vi "Main Loop.vi"(8 "error in (no error)":errorcluster, 10 "Chart Notifier":refnum<notifier>, 11 "Message Queues":T1) -> (0 "error out":errorcluster)   [LabVIEW 2018, in "TCU Module.lvlib" / "TCU Module Engine.lvlib"]
uses:
  TCU Module Engine.lvlib
  All Message Queues.ctl
  support/Message Queue/Message Cluster.ctl
  TCU State Cluster.ctl
  State Enum.ctl
  TCU Module Settings Cluster.ctl
  Output Devices.ctl
  Huber TCU/Huber Settings.ctl
  Lauda Integral XT-150 TCU/Lauda Settings.ctl
  Julabo Type 1 TCU/Julabo Type 1 TCU Folder/Julabo FP-50 Settings.ctl
  Huber Unistat 410 TCU/Huber Unistat 410 Settings.ctl
  TCU Module Display.ctl
  <vilib>/Platform/TimedLoop/XDataNode/timing_clust.ctl
  <vilib>/Platform/TimedLoop/XDataNode/nitl_modes.ctl
  <vilib>/Platform/TimedLoop/XDataNode/wakeup.ctl
  Tag VIs/Tag FGV Operation Enum.ctl
  TCU Module Config Cluster.ctl
  <vilib>/Utility/miscctls.llb/LVPoint32TypeDef.ctl
  support/Message Queue/Enqueue Message (Single).vi
  <vilib>/Platform/TimedLoop/XDataNode/XDataNode.xnode
  support/Message Queue/Message Queue.lvlib
  <vilib>/Platform/TimedLoop/XDataNode/XDNodeRunTimeDep.lvlib
  TCU Module.lvlib
  Shared Variables/Dynamic Shared Variables.lvlib
  Huber TCU/Huber Ministat 230 TCU.lvlib
  Lauda Integral XT-150 TCU/Lauda TCU.lvlib
  Julabo Type 1 TCU/Julabo Type 1 TCU Folder/Julabo Type FP-50 TCU.lvlib
  Huber Unistat 410 TCU/Huber Unistat 410 TCU.lvlib
  support/Support Library.lvlib
panel:
  out "Period (s)":dbl format="%_4g"
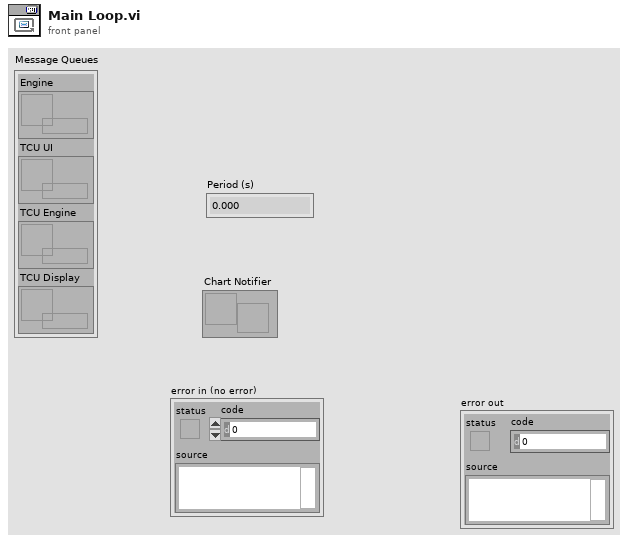
[diagram p1: front panel]
types:
  T1 = typedef "TCU Module.lvlib/All Message Queues.ctl" = cluster{"Engine":refnum<queue>, "TCU UI":refnum<queue>, "TCU Engine":refnum<queue>, "TCU Display":refnum<queue>}
  T2 = typedef "XDNodeRunTimeDep.lvlib/timing_clust.ctl" = cluster{"Expected End [f-1]":u64, "Actual End [f-1]":u64, "Finished Late? [f-1]":bool, "Expected End [i-1]":u64, "Actual End [i-1]":u64, "Finished Late? [i-1]":bool, "Expected Start [i]":u64, "Actual Start [i]":u64, "Expected Start [f]":u64, "Actual Start [f]":u64, "Source Name":string, "Structure Name":string, "Period":i64, "Deadline":i64, "Offset":i64, "Start":i64, "Priority":i32, "Timeout":i32, "Mode":T3, "Wakeup Reason":T4, "Error":errorcluster, "Source Type":string, "Secondary Source Type":string, "Global End Time":u64, "Global Start Time":u64, "Frame Duration":u64, "Iteration Duration":u64, "Assigned CPU":i32, "I/O Scan Engine Mode":u32}
  T3 = typedef "XDNodeRunTimeDep.lvlib/nitl_modes.ctl" = enum32{"No Change", "Process missed periods, maintain original phase", "Discard missed periods, maintain original phase", "Process missed periods, ignore original phase", "Discard missed periods, ignore original phase"}
  T4 = typedef "XDNodeRunTimeDep.lvlib/wakeup.ctl" = enum32{"Normal", "Aborted", "Asynchronous wakeup", "Timing source error", "Timed loop error", "Timeout"}
  T5 = cluster{"enable? (F)":bool, "name":string, "alarm on":bool, "priority":u32, "ack type":enum16{"Auto", "User", "None", "Each Occurrence"}, "area":string, "description":string, "log? (T)":bool}
  T6 = typedef "Tag FGV Operation Enum.ctl" = enum16{"Init", "Set Notification Queue", "Create Tag", "Commit", "Write Tag (Numeric)", "Write Tag (Boolean)", "Read All Tags", "Read One Tag", "Delete Tag Category", "Set Alarm Parameters (Numeric)", "Set Alarm Parameters (Boolean)", "Enable All Alarms", "Disable All Alarms", "Delete All Tags", "Read Alarms", "Ack Alarm", "Read Alarm Parameters (Numeric)", "Read Alarm Parameters (Boolean)"}
  T7 = enum32{"u32BitField", "bool", "double", "string", "int8", "uint8", "int16", "uint16", "int32", "uint32", "int64", "uint64", "single", "double waveform", "int16 waveform", "array of boolean", "array of int8", "array of uint8", "array of int16", "array of uint16", "array of int32", "array of uint32", "array of int64", "array of uint64", "array of single", "array of double", "array of double waveform", "array of int16 waveform", "array of string", "variant", "timestamp", "fixed point", "custom"}
  T8 = typedef "TCU Module.lvlib/TCU Module Engine.lvlib/State Enum.ctl" = enum16{"Measuring", "Idle", "Paused"}
  T9 = typedef "TCU Module.lvlib/TCU Module Config Cluster.ctl" = cluster{"GUID":string, "Drop Coords":T10, "Process Name":string, "Queue Name":string, "Settings":T11, "Load Count":i32, "Power Level Changed":bool}
  T10 = typedef "LVPoint32TypeDef.ctl" = cluster{"Horizontal":i32, "Vertical":i32}
  T11 = typedef "TCU Module.lvlib/TCU Module Settings Cluster.ctl" = cluster{"Cycle Period":dbl, "Setpoint Entry":dbl, "Output Device":T12, "Huber Ministat 230 Settings":T13, "Lauda Settings":T14, "Julabo FP-50 Settings":T15, "Internal Control?":bool, "Huber Unistat 410 Settings":T16}
  T12 = typedef "Output Devices.ctl" = enum16{"Default", "Huber Ministat 230", "Huber Unistat 410", "Lauda XT-150", "Julabo FP-50"}
  T13 = typedef "Huber Ministat 230 TCU.lvlib/Huber Settings.ctl" = cluster{"VISA resource name":refnum<visa-resource-name>, "Simulated?":bool}
  T14 = typedef "Lauda TCU.lvlib/Lauda Settings.ctl" = cluster{"VISA resource name":refnum<visa-resource-name>, "Simulated?":bool, "Pump Power":i32}
  T15 = typedef "Julabo Type FP-50 TCU.lvlib/Julabo FP-50 Settings.ctl" = cluster{"VISA resource name":refnum<visa-resource-name>, "Simulated?":bool, "Pump Power":i32}
  T16 = typedef "Huber Unistat 410 TCU.lvlib/Huber Unistat 410 Settings.ctl" = cluster{"VISA resource name":refnum<visa-resource-name>, "Simulated?":bool}
  T17 = typedef "TCU Module.lvlib/TCU Module Display.ctl" = cluster{"TCU On?":bool, "Cycle Period":dbl, "Current TCU Temp":dbl}
  T18 = typedef "TCU Module.lvlib/TCU Module Engine.lvlib/TCU State Cluster.ctl" = cluster{"State":T8, "Start Time":timestamp, "Configuration":T11, "Current Time":timestamp, "First Iteration":bool, "Data":cluster{"TCU Speed":dbl, "Temperature":dbl}, "Process Name":string, "TCU On?":bool, "Output Error":bool, "Start Log":bool, "Power Level Changed":bool}
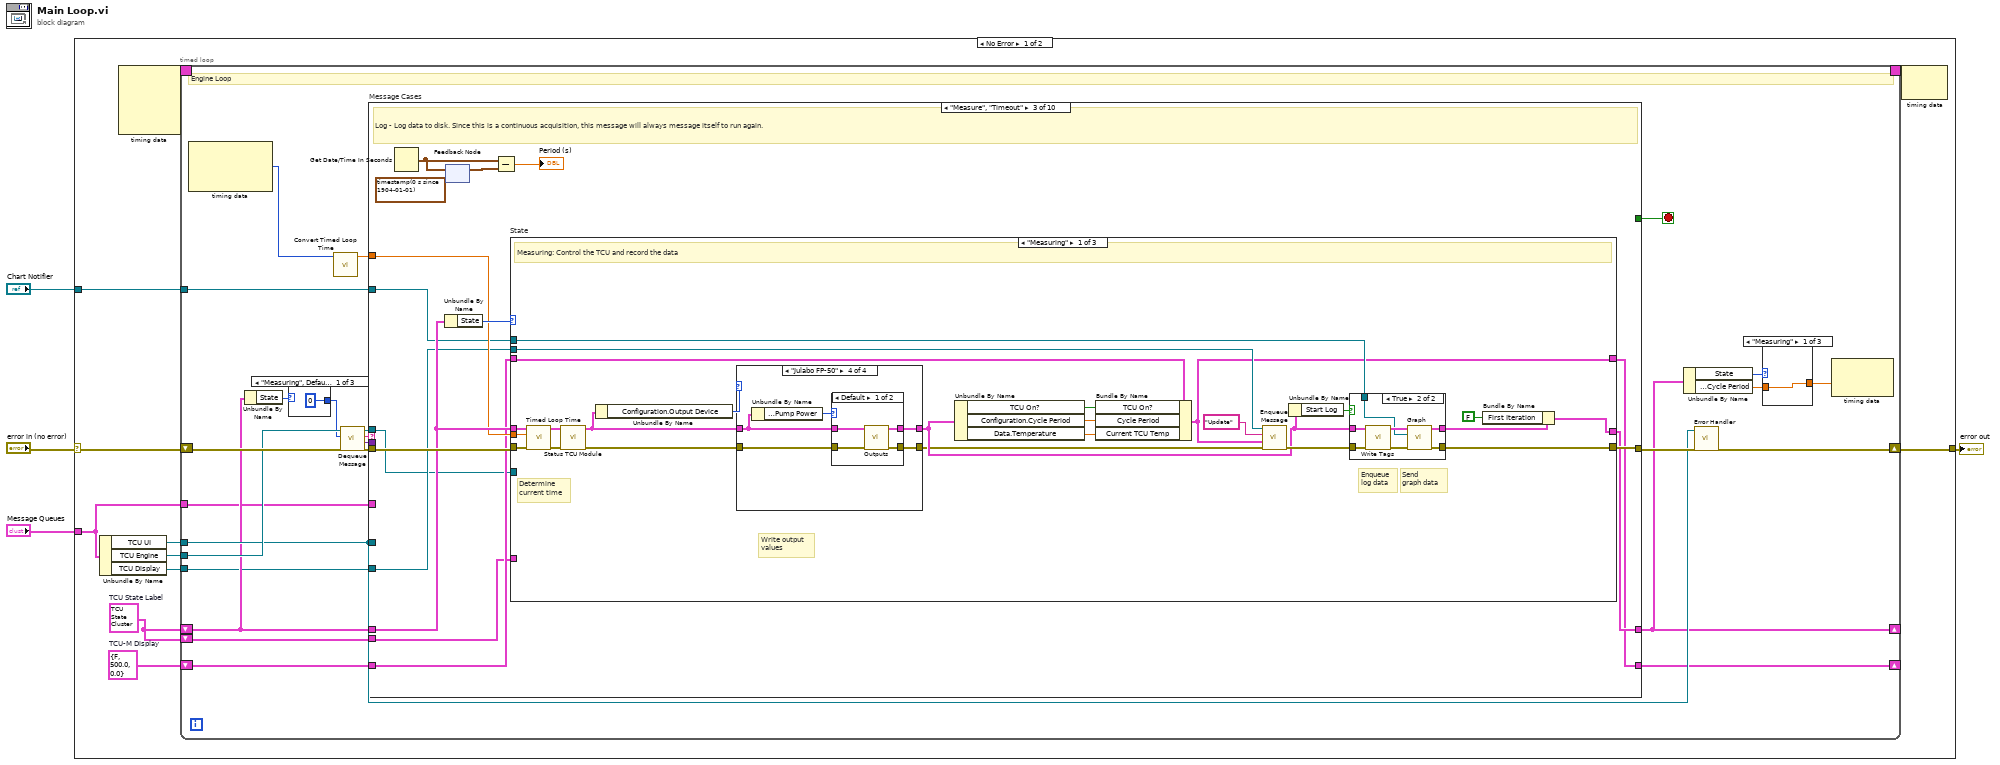
[diagram p0: block diagram]
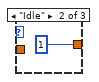
[diagram p2: hidden frame]
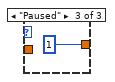
[diagram p3: hidden frame]
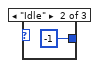
[diagram p4: hidden frame]
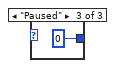
[diagram p5: hidden frame]
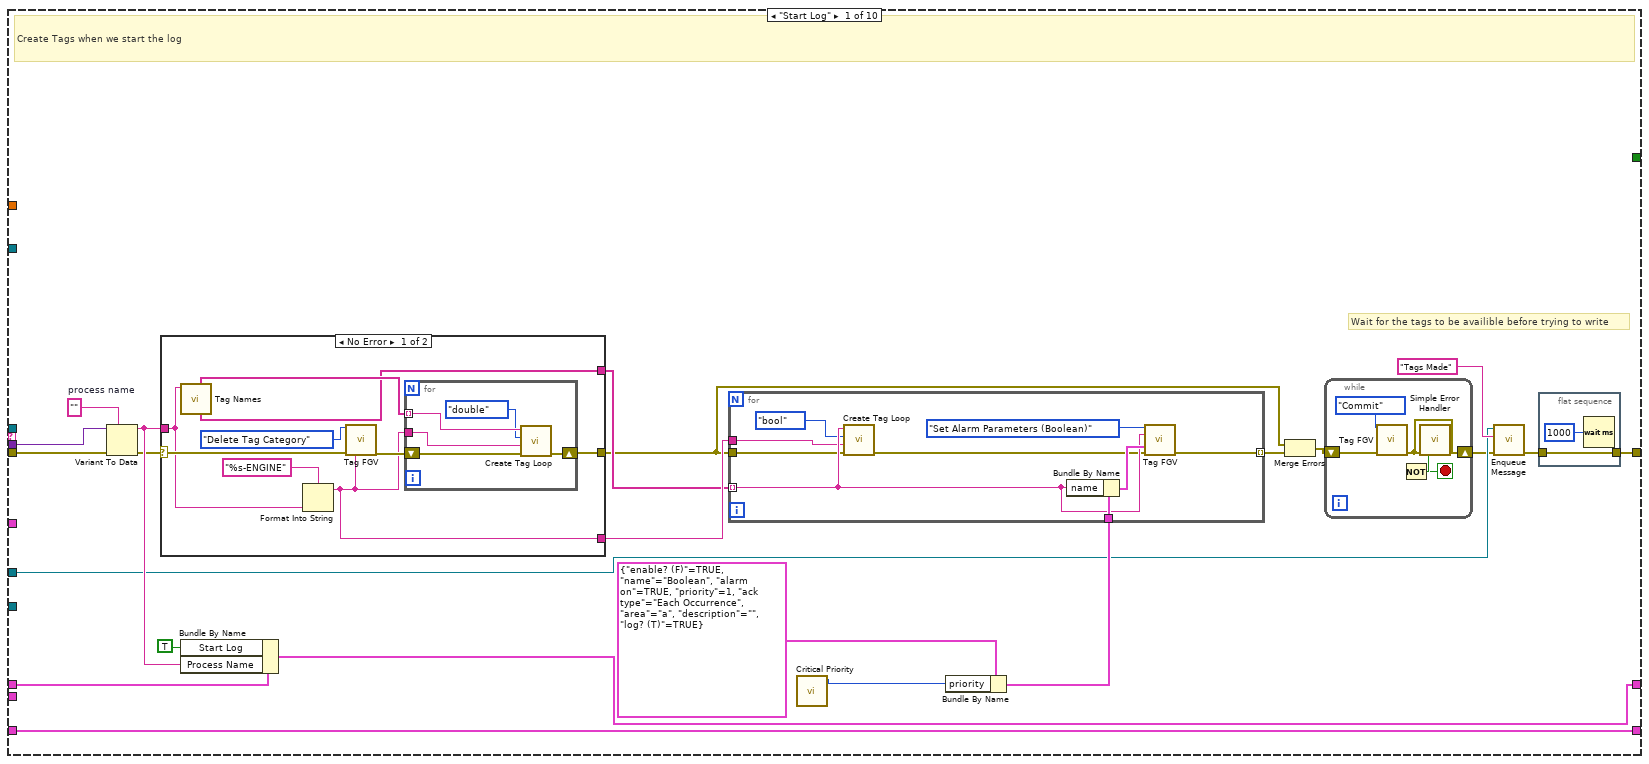
[diagram p6: hidden frame]
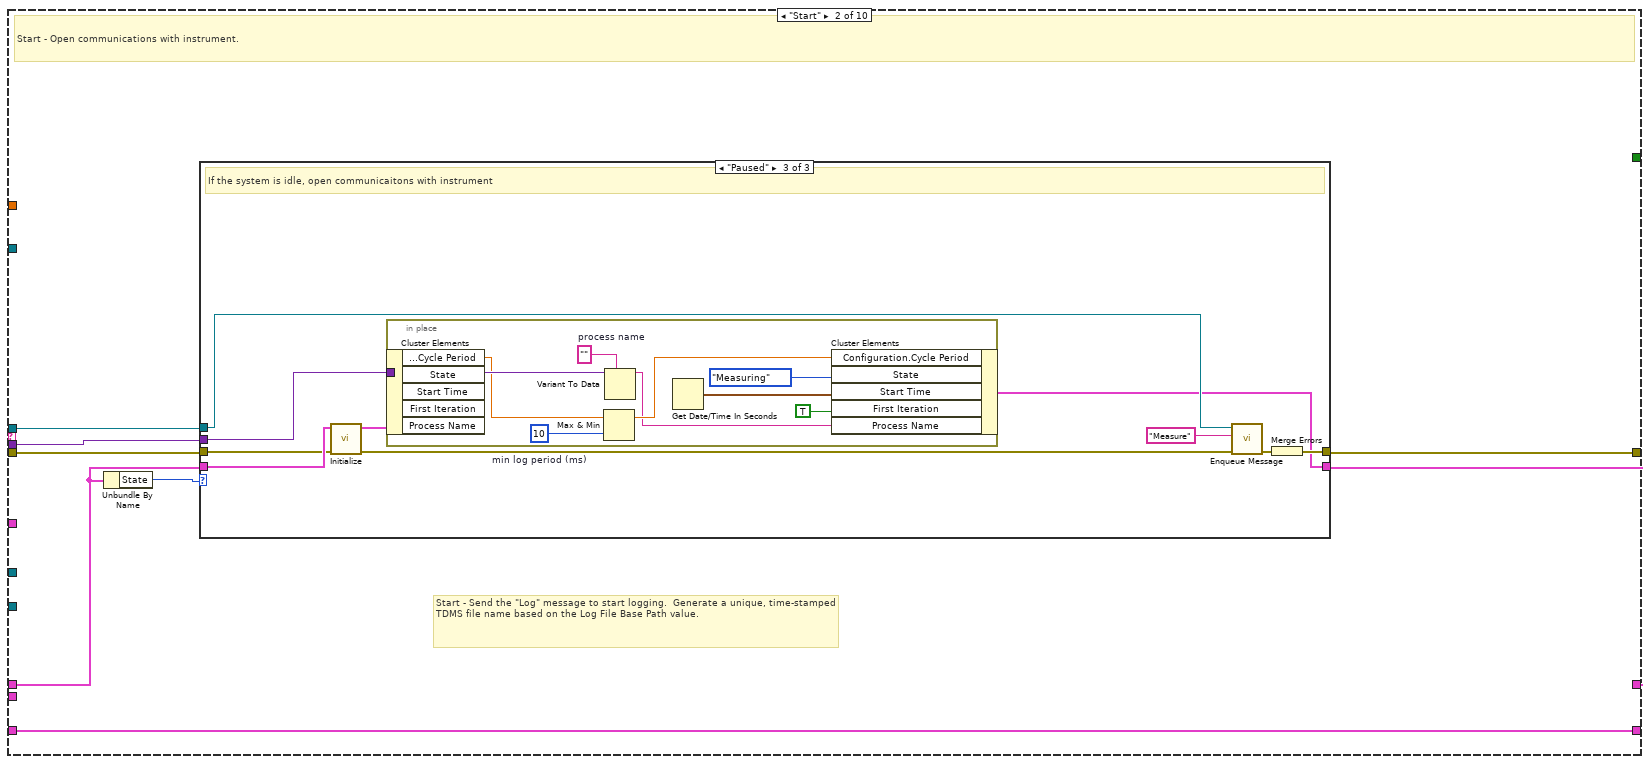
[diagram p8: hidden frame]
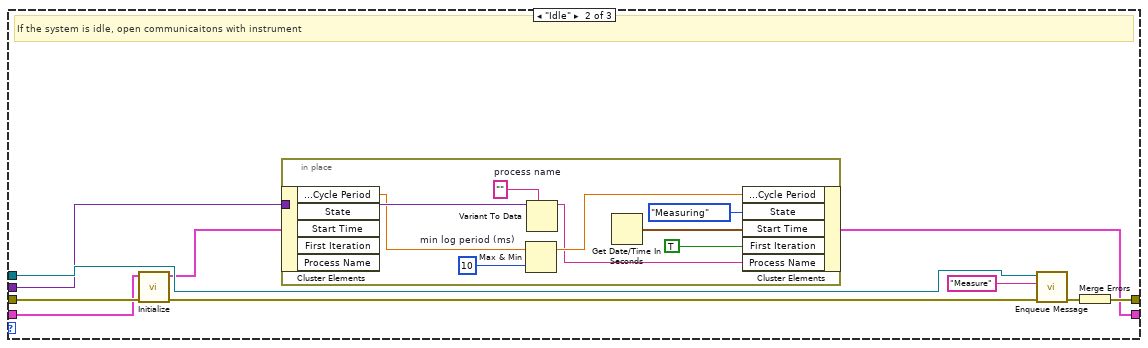
[diagram p10: hidden frame]
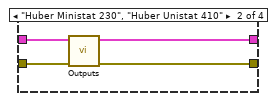
[diagram p12: hidden frame]
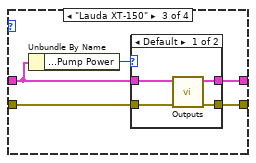
[diagram p13: hidden frame]
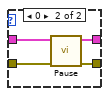
[diagram p14: hidden frame]
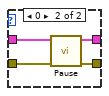
[diagram p15: hidden frame]
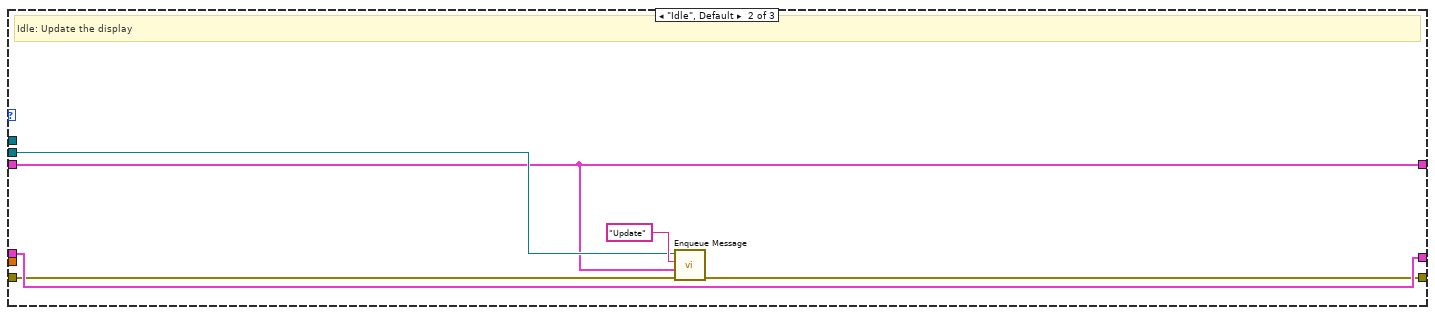
[diagram p17: hidden frame]
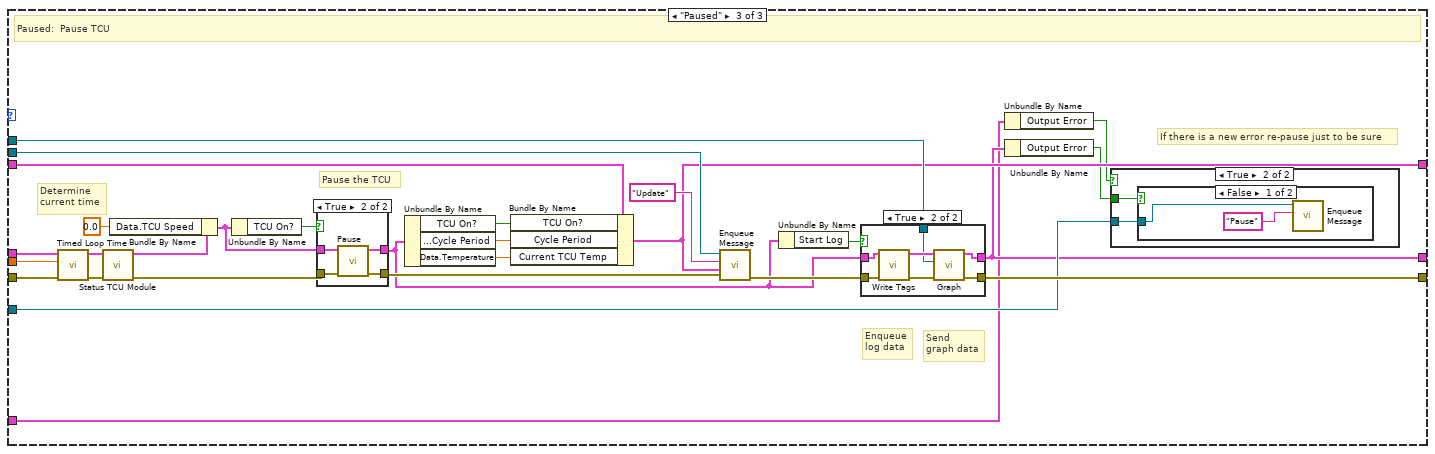
[diagram p18: hidden frame]
diagram:
  n1 = case shown="No Error" "error in (no error)" {
    selector: "error in (no error)" -> [w14 w373]
    tunnel: "Message Queues" -> [w10 _]
    tunnel: [w15 w373] -> w3
    tunnel: "Chart Notifier" -> [w8 _]
    frame No Error {
      w6 = T17 {"TCU On?"=FALSE, "Cycle Period"=500.0, "Current TCU Temp"=0.0}  # TCU-M Display
      w5 = T18 {"State"=enum."Idle", "Start Time"=timestamp(0 s since 1904-01-01), "Configuration"={"Cycle Period"=0.0, "Setpoint Entry"=0.0, "Output Device"=enum."Default", "Huber Ministat 230 Settings"={"VISA resource name"="", "Simulated?"=FALSE}, "Lauda Settings"={"VISA resource name"="", "Simulated?"=FALSE, "Pump Power"=2}, "Julabo FP-50 Settings"={"VISA resource name"="", "Simulated?"=FALSE, "Pump Power"=2}, "Internal Control?"=FALSE, "Huber Unistat 410 Settings"={"VISA resource name"="", "Simulated?"=FALSE}}, "Current Time"=timestamp(0 s since 1904-01-01), "First Iteration"=FALSE, "Data"={"TCU Speed"=0.0, "Temperature"=0.0}, "Process Name"="", "TCU On?"=FALSE, "Output Error"=FALSE, "Start Log"=FALSE, "Power Level Changed"=FALSE}  # TCU State Label
      n2 = Unbundle By Name(w10) -> ("TCU UI"=w13:refnum<queue>, "TCU Engine"=w9:refnum<queue>, "TCU Display"=w7:refnum<queue>)
      n3 = node-c288() -> (w12:T2)  [unwired: 4 in]
      n4 = timed-loop {
        tunnel: w9 -> [w34]
        shift-right: [w27] -> _
        shift-left: w5 -> [w30]
        shift-right: [w32] -> w15
        shift-left: w14 -> [w39]
        tunnel: w13 -> [w31]
        timing: w12 -> [_]
        timing-out: [_] -> w11
        tunnel: w10 -> [w21]
        tunnel: w8 -> [w20]
        tunnel: w7 -> [w19]
        shift-right: [w18] -> _
        shift-left: w6 -> [w17]
        shift-left: w5 -> [w16]
        stop <- w40 stop-if-true
        # "Engine Loop"
        n5 = node-c288() -> (w23:i64)  [unwired: 1 in, 2 out]
        n6 = Unbundle By Name(w30) -> ("State"=w29:T8)
        n7 = case shown="\"Measuring\", Default" w29 {
          tunnel: [0 ("timeout in ms (-1)") -1 ("timeout in ms (-1)") 0 ("timeout in ms (-1)")] -> w28
          frame "Measuring", Default {
          }
          frame "Idle" {
          }
          frame "Paused" {
          }
        }
        n8 = call "Convert Timed Loop Time.vi"("Actual Start [i]"=w23) -> ("ET since start (s)"=w22:dbl)  [unwired: 10 in]
        n9 = call "Dequeue Message.vi"("error in (no error)"=w39, "timeout in ms (-1)"=w28, "Message Queue"=w34) -> ("error out"=w38:errorcluster, "Message Data"=w36:variant, "Message"=w37:string, "dup Message Queue"=w35:refnum<queue>)  [unwired: 5 in]
        n10 = case "Message Cases" shown="\"Measure\", \"Timeout\"" w37 {
          selector: w37 -> [_ _ _ _ _ _ _ _ _ w363]
          tunnel: w35 -> [_ w111 w155 _ _ _ w345 _ _ _]
          tunnel: w38 -> [w71 w110 w166 w296 w316 w339 w348 w355 w362 _]
          tunnel: [w53 w112 w167 w289 w309 w335 w350 w353 w361 w364] -> w33
          tunnel: w30 -> [w70 w106 w164 w293 w314 w337 w343 w354 w359 w370]
          tunnel: [w69 w109 w165 w292 w313 w336 w343 w354 w356 w370] -> w27
          tunnel: [_ _ _ _ _ _ TRUE _ _ _] -> w40
          tunnel: w36 -> [w72 w107 _ _ _ w340 _ _ _ _]
          tunnel: w31 -> [w57 _ _ w295 _ _ w349 _ _ _]
          tunnel: w22 -> [_ _ w163 _ _ _ _ _ _ _]
          tunnel: w21 -> [_ _ _ _ _ _ _ _ _ _]
          tunnel: w20 -> [_ _ w159 _ _ _ _ _ _ _]
          tunnel: w19 -> [_ _ w158 w288 w311 _ _ _ _ _]
          tunnel: w17 -> [w73 w105 w157 w287 w308 w338 w341 w352 w360 w369]
          tunnel: [w73 w105 w156 w287 w308 w338 w341 w352 w360 w369] -> w18
          tunnel: w16 -> [_ _ w154 _ _ _ _ _ _ _]
          frame "Start Log" {
            w68 = ""  # process name
            # "Wait for the tags to be availible before trying to write"
            # "Create Tags when we start the log"
            n11 = Variant To Data(error in=w71, type=w68, Variant=w72) -> (data=w67:string, error out=w66:errorcluster)
            n12 = case shown="No Error" w66 {
              selector: w66 -> [w95 w104]
              tunnel: [w98 w104] -> w52
              tunnel: w67 -> [w93 _]
              tunnel: [w91 _] -> w62
              tunnel: [w90 _] -> w61
              frame No Error {
                n13 = call "Tag Names.vi"("Process Name"=w93) -> ("All Boolean Tags"=w90:string[], "All  Numeric Tags"=w92:string[])  [unwired: 8 in, 1 out]
                n14 = Format Into String(format string="%s-ENGINE", w93) -> (resulting string=w91:string)  [unwired: 2 in, 1 out]
                n15 = call "Tag FGV.vi"("Operation"=Tag_FGV_Operation_Enum."Delete Tag Category", "error in (no error)"=w95, "Tag Category"=w91) -> ("error out"=w94:errorcluster)  [unwired: 5 in, 7 out]
                n16 = for {
                  shift-right: [w99] -> w98
                  shift-left: w94 -> [w102]
                  tunnel: w91 -> [w101]
                  tunnel: w92 -> [w103] mode=indexing
                  n17 = call "Create Tag Loop.vi"("error in (no error)"=w102, "Tag Category"=w101, "data type"=T7."double", "Tag Name"=w103) -> ("error out"=w99:errorcluster)  [unwired: 7 in]
                }
              }
              frame Error {
              }
            }
            n18 = Bundle By Name(cluster=w70, "Start Log"=TRUE, "Process Name"=w67) -> (w69:T18)
            n19 = call "Critical Priority.vi"() -> ("critical priority"=w65:i32)  [unwired: 11 in]
            n20 = Bundle By Name(cluster=T5 {"enable? (F)"=TRUE, "name"="Boolean", "alarm on"=TRUE, "priority"=1, "ack type"=enum."Each Occurrence", "area"="a", "description"="", "log? (T)"=TRUE} ("Boolean alarm settings"), "priority"=w65) -> (w63:T5)
            n21 = for {
              tunnel: w63 -> [w89]
              tunnel: [w88] -> w60 mode=indexing
              tunnel: w61 -> [w85] mode=indexing
              tunnel: w52 -> [w82]
              tunnel: w62 -> [w83]
              n22 = call "Create Tag Loop.vi"("error in (no error)"=w82, "Tag Category"=w83, "data type"=T7."bool", "Tag Name"=w85) -> ("error out"=w81:errorcluster)  [unwired: 7 in]
              n23 = Bundle By Name(cluster=w89, "name"=w85) -> (w87:T5)
              n24 = call "Tag FGV.vi"("Operation"=Tag_FGV_Operation_Enum."Set Alarm Parameters (Boolean)", "Tag Name"=w85, "Data"=w87, "error in (no error)"=w81) -> ("error out"=w88:errorcluster)  [unwired: 4 in, 7 out]
            }
            n25 = Merge Errors(w52, w60) -> (w56:errorcluster)
            n26 = while {
              shift-right: [w78] -> w55
              shift-left: w56 -> [w79]
              stop <- w76 stop-if-true
              n27 = call "Tag FGV.vi"("Operation"=Tag_FGV_Operation_Enum."Commit", "error in (no error)"=w79) -> ("error out"=w78:errorcluster)  [unwired: 6 in, 7 out]
              n28 = call <vilib>:"Simple Error Handler.vi"("error in (no error)"=w78) -> ("error?"=w77:bool)  [unwired: 4 in, 4 out]
              n29 = Not(x=w77) -> (.not. x?=w76:bool)
            }
            n30 = call-poly "Enqueue Message.vi"("error in (no error)"=w55, "Message"="Tags Made", "Message Queue"=w57) -> ("error out"=w54:errorcluster)  [unwired: 7 in, 1 out]
            n31 = flat-sequence {
              tunnel: w54 -> [w74]
              tunnel: [w74] -> w53
              frame #0 {
                n32 = Wait (ms)(milliseconds to wait=u32 1000) -> ()  [unwired: 1 out]
              }
            }
          }
          frame "Start" {
            # "Start - Send the \"Log\" message to start logging.  Generate a unique, time-stamped TDMS file name based on the Log File Base Path value."
            # "Start - Open communications with instrument."
            n33 = Unbundle By Name(w106) -> ("State"=w108:T8)
            n34 = case shown="\"Paused\"" w108 {
              tunnel: [w113 w124 w143] -> w112
              tunnel: w111 -> [_ w121 w140]
              tunnel: w110 -> [w113 w120 w137]
              tunnel: w106 -> [w114 w119 w138]
              tunnel: [w114 w115 w134] -> w109
              tunnel: w107 -> [_ w118 w139]
              frame "Measuring", Default {
                # "The system is already running. Ignore the \"Start\" message."
              }
              frame "Idle" {
                # "If the system is idle, open communicaitons with instrument"
                n35 = call "Initialize.vi"("error in (no error)"=w120, "State in"=w119) -> ("error out"=w117:errorcluster, "State out"=w116:T18)  [unwired: 8 in]
                n36 = in-place {
                  in-place-border: w118 -> [w131]
                  w132 = ""  # process name
                  w133 = 10  # min log period (ms)
                  n37 = in-place-cluster #1(w116) -> ("Configuration.Cycle Period"=w130:dbl)  [unwired: 4 out]
                  n38 = Max & Min(x=w130, y=w133) -> (max(x,y)=w129:dbl)  [unwired: 1 out]
                  n39 = Variant To Data(type=w132, Variant=w131) -> (data=w125:string)  [unwired: 1 in, 1 out]
                  n40 = Get Date/Time In Seconds() -> (seconds since 1Jan1904=w127:timestamp)
                  n41 = in-place-cluster #1("Configuration.Cycle Period"=w129, "State"=State_Enum."Measuring", "Start Time"=w127, "First Iteration"=TRUE, "Process Name"=w125) -> (w115:T18)
                }
                n42 = call-poly "Enqueue Message.vi"("error in (no error)"=w117, "Message"="Measure", "Message Queue"=w121) -> ("error out"=w122:errorcluster)  [unwired: 7 in, 1 out]
                n43 = Merge Errors(w122) -> (w124:errorcluster)
              }
              frame "Paused" {
                # "If the system is idle, open communicaitons with instrument"
                n44 = call "Initialize.vi"("error in (no error)"=w137, "State in"=w138) -> ("error out"=w136:errorcluster, "State out"=w135:T18)  [unwired: 8 in]
                n45 = in-place {
                  in-place-border: w139 -> [w150]
                  w151 = ""  # process name
                  w152 = 10  # min log period (ms)
                  n46 = in-place-cluster #2(w135) -> ("Configuration.Cycle Period"=w149:dbl)  [unwired: 4 out]
                  n47 = Max & Min(x=w149, y=w152) -> (max(x,y)=w148:dbl)  [unwired: 1 out]
                  n48 = Variant To Data(type=w151, Variant=w150) -> (data=w144:string)  [unwired: 1 in, 1 out]
                  n49 = Get Date/Time In Seconds() -> (seconds since 1Jan1904=w146:timestamp)
                  n50 = in-place-cluster #2("Configuration.Cycle Period"=w148, "State"=State_Enum."Measuring", "Start Time"=w146, "First Iteration"=TRUE, "Process Name"=w144) -> (w134:T18)
                }
                n51 = call-poly "Enqueue Message.vi"("error in (no error)"=w136, "Message"="Measure", "Message Queue"=w140) -> ("error out"=w141:errorcluster)  [unwired: 7 in, 1 out]
                n52 = Merge Errors(w141) -> (w143:errorcluster)
              }
            }
          }
          frame "Measure", "Timeout" {
            # "Log - Log data to disk. Since this is a continuous acquisition, this message will always message itself to run again."
            n53 = Get Date/Time In Seconds() -> (seconds since 1Jan1904=w161:timestamp)
            n54 = Unbundle By Name(w164) -> ("State"=w168:T8)
            n55 = feedback-in #3(w161) -> ()
            n56 = feedback #3(timestamp(0 s since 1904-01-01) ("seconds since 1Jan1904")) -> (w162:timestamp)
            n57 = Subtract(x=w161, y=w162) -> (x-y=→"Period (s)":dbl)
            n58 = case "State" shown="\"Measuring\"" w168 {
              tunnel: w166 -> [w191 w235 w261]
              tunnel: w164 -> [w190 w239 w262]
              tunnel: [w192 w234 w255] -> w167
              tunnel: [w187 w239 w249] -> w165
              tunnel: w163 -> [w189 _ w266]
              tunnel: w159 -> [w185 _ w267]
              tunnel: w158 -> [w184 w237 w263]
              tunnel: w157 -> [w182 w236 w264]
              tunnel: [w180 w236 w254] -> w156
              tunnel: w155 -> [_ _ w250]
              tunnel: w154 -> [_ _ w246]
              frame "Measuring" {
                # "Determine\ncurrent time"
                # "Send\ngraph data"
                # "Enqueue\nlog data"
                # "Write output\nvalues"
                # "Measuring: Control the TCU and record the data"
                n59 = call "Timed Loop Time.vi"("error in (no error)"=w191, "ET since start (s)"=w189, "State in"=w190) -> ("error out"=w179:errorcluster, "State out"=w178:T18)  [unwired: 7 in]
                n60 = call "Status TCU Module.vi"("error in (no error)"=w179, 11:w178) -> ("error out"=w171:errorcluster, "State out"=w172:T18)  [unwired: 8 in]
                n61 = Unbundle By Name(w172) -> ("Configuration.Output Device"=w173:T12)
                n62 = case shown="\"Julabo FP-50\"" w173 {
                  tunnel: w172 -> [w194 w198 w203 w215]
                  tunnel: w171 -> [w193 w197 w200 w214]
                  tunnel: [w194 w195 w201 w212] -> w170
                  tunnel: [w193 w196 w202 w213] -> w169
                  frame Default {
                  }
                  frame "Huber Ministat 230", "Huber Unistat 410" {
                    n63 = call "Outputs.vi"("error in (no error)"=w197, "State in"=w198) -> ("error out"=w196:errorcluster, "State out"=w195:T18)  [unwired: 8 in]
                  }
                  frame "Lauda XT-150" {
                    n64 = Unbundle By Name(w203) -> ("Configuration.Lauda Settings.Pump Power"=w199:i32)
                    n65 = case shown="Default" w199 {
                      tunnel: w200 -> [w207 w210]
                      tunnel: [w206 w209] -> w202
                      tunnel: w203 -> [w205 w211]
                      tunnel: [w204 w208] -> w201
                      frame Default {
                        n66 = call "Outputs.vi"("error in (no error)"=w207, "State in"=w205) -> ("error out"=w206:errorcluster, "State out"=w204:T18)  [unwired: 8 in]
                      }
                      frame 0 {
                        n67 = call "Pause.vi"("error in (no error)"=w210, "State in"=w211) -> ("error out"=w209:errorcluster, "State out"=w208:T18)  [unwired: 8 in]
                      }
                    }
                  }
                  frame "Julabo FP-50" {
                    n68 = Unbundle By Name(w215) -> ("Configuration.Julabo FP-50 Settings.Pump Power"=w216:i32)
                    n69 = case shown="Default" w216 {
                      tunnel: w214 -> [w220 w223]
                      tunnel: [w219 w222] -> w213
                      tunnel: w215 -> [w218 w224]
                      tunnel: [w217 w221] -> w212
                      frame Default {
                        n70 = call "Outputs.vi"("error in (no error)"=w220, "State in"=w218) -> ("error out"=w219:errorcluster, "State out"=w217:T18)  [unwired: 8 in]
                      }
                      frame 0 {
                        n71 = call "Pause.vi"("error in (no error)"=w223, "State in"=w224) -> ("error out"=w222:errorcluster, "State out"=w221:T18)  [unwired: 8 in]
                      }
                    }
                  }
                }
                n72 = Unbundle By Name(w170) -> ("TCU On?"=w181:bool, "Configuration.Cycle Period"=w176:dbl, "Data.Temperature"=w175:dbl)
                n73 = Bundle By Name(cluster=w182, "TCU On?"=w181, "Cycle Period"=w176, "Current TCU Temp"=w175) -> (w180:T17)
                n74 = call-poly "Enqueue Message.vi"("error in (no error)"=w169, "Message Data"=w180, "Message"="Update", "Message Queue"=w184) -> ("error out"=w177:errorcluster)  [unwired: 6 in, 1 out]
                n75 = Unbundle By Name(w170) -> ("Start Log"=w174:bool)
                n76 = case shown="True" w174 {
                  tunnel: [w225 w231] -> w192
                  tunnel: [w226 w230] -> w188
                  tunnel: w185 -> [_ w229]
                  tunnel: w170 -> [w226 w228]
                  tunnel: w177 -> [w225 w227]
                  frame False {
                  }
                  frame True {
                    n77 = call "Write Tags.vi"("error in (no error)"=w227, "State in"=w228) -> ("error out"=w232:errorcluster, "State out"=w233:T18)  [unwired: 8 in]
                    n78 = call "Graph.vi"("error in (no error)"=w232, "notifier out"=w229, "State in"=w233) -> ("error out"=w231:errorcluster, "State out"=w230:T18)  [unwired: 7 in]
                  }
                }
                n79 = Bundle By Name(cluster=w188, "First Iteration"=FALSE) -> (w187:T18)
              }
              frame "Idle", Default {
                # "Idle: Update the display"
                n80 = call-poly "Enqueue Message.vi"("error in (no error)"=w235, "Message Data"=w236, "Message"="Update", "Message Queue"=w237) -> ("error out"=w234:errorcluster)  [unwired: 6 in, 1 out]
              }
              frame "Paused" {
                # "If there is a new error re-pause just to be sure"
                # "Determine\ncurrent time"
                # "Pause the TCU"
                # "Send\ngraph data"
                # "Enqueue\nlog data"
                # "Paused:  Pause TCU"
                n81 = call "Timed Loop Time.vi"("error in (no error)"=w261, "ET since start (s)"=w266, "State in"=w262) -> ("error out"=w259:errorcluster, "State out"=w260:T18)  [unwired: 7 in]
                n82 = call "Status TCU Module.vi"("error in (no error)"=w259, 11:w260) -> ("error out"=w258:errorcluster, "State out"=w242:T18)  [unwired: 8 in]
                n83 = Bundle By Name(cluster=w242, "Data.TCU Speed"=0.0) -> (w240:T18)
                n84 = Unbundle By Name(w240) -> ("TCU On?"=w243:bool)
                n85 = case shown="True" w243 {
                  tunnel: w240 -> [w278 w282]
                  tunnel: w258 -> [w277 w281]
                  tunnel: [w277 w280] -> w257
                  tunnel: [w278 w279] -> w245
                  frame False {
                  }
                  frame True {
                    n86 = call "Pause.vi"("error in (no error)"=w281, "State in"=w282) -> ("error out"=w280:errorcluster, "State out"=w279:T18)  [unwired: 8 in]
                  }
                }
                n87 = Unbundle By Name(w245) -> ("TCU On?"=w253:bool, "Configuration.Cycle Period"=w252:dbl, "Data.Temperature"=w251:dbl)
                n88 = Bundle By Name(cluster=w264, "TCU On?"=w253, "Cycle Period"=w252, "Current TCU Temp"=w251) -> (w254:T17)
                n89 = call-poly "Enqueue Message.vi"("error in (no error)"=w257, "Message Data"=w254, "Message"="Update", "Message Queue"=w263) -> ("error out"=w256:errorcluster)  [unwired: 6 in, 1 out]
                n90 = Unbundle By Name(w245) -> ("Start Log"=w244:bool)
                n91 = case shown="True" w244 {
                  tunnel: w267 -> [_ w274]
                  tunnel: w256 -> [w268 w273]
                  tunnel: [w268 w272] -> w255
                  tunnel: w245 -> [w269 w271]
                  tunnel: [w269 w270] -> w249
                  frame False {
                  }
                  frame True {
                    n92 = call "Write Tags.vi"("error in (no error)"=w273, "State in"=w271) -> ("error out"=w276:errorcluster, "State out"=w275:T18)  [unwired: 8 in]
                    n93 = call "Graph.vi"("error in (no error)"=w276, "notifier out"=w274, "State in"=w275) -> ("error out"=w272:errorcluster, "State out"=w270:T18)  [unwired: 7 in]
                  }
                }
                n94 = Unbundle By Name(w246) -> ("Output Error"=w247:bool)
                n95 = Unbundle By Name(w249) -> ("Output Error"=w248:bool)
                n96 = case shown="True" w247 {
                  tunnel: w248 -> [_ w284]
                  tunnel: w250 -> [_ w283]
                  frame False {
                  }
                  frame True {
                    n97 = case shown="False" w284 {
                      tunnel: w283 -> [w286 _]
                      frame False {
                        n98 = call-poly "Enqueue Message.vi"("Message"="Pause", "Message Queue"=w286) -> ()  [unwired: 8 in, 2 out]
                      }
                      frame True {
                      }
                    }
                  }
                }
              }
            }
          }
          frame "Stop" {
            # "Stop - Stop the TCU and Close the Connections"
            n99 = Unbundle By Name(w293) -> ("State"=w294:T8)
            n100 = case shown="\"Measuring\", Default" w294 {
              tunnel: [w301 w307] -> w290
              tunnel: w296 -> [w298 w307]
              tunnel: w295 -> [w305 _]
              tunnel: w293 -> [w299 w306]
              tunnel: [w303 w306] -> w292
              frame "Measuring", Default {
                # "If the system is logging, stop logging."
                n101 = call "Close.vi"("error in (no error)"=w298, "State in"=w299) -> ("error out"=w297:errorcluster, "State out"=w300:T18)  [unwired: 8 in]
                n102 = Bundle By Name(cluster=w300, "State"=State_Enum."Idle") -> (w303:T18)
                n103 = call-poly "Enqueue Message.vi"("error in (no error)"=w297, "Message"="Logging Stopped", "Message Queue"=w305) -> ("error out"=w301:errorcluster)  [unwired: 7 in, 1 out]
              }
              frame "Idle" {
                # "The system is already idle. Ignore the \"Stop\" message."
              }
            }
            n104 = call-poly "Enqueue Message.vi"("error in (no error)"=w290, "Message Data"=w287, "Message"="Update", "Message Queue"=w288) -> ("error out"=w289:errorcluster)  [unwired: 6 in, 1 out]
          }
          frame "Pause" {
            # "Pause: Stop the TCU but don't disconnect"
            n105 = Unbundle By Name(w314) -> ("State"=w315:T8)
            n106 = case shown="\"Measuring\", Default" w315 {
              tunnel: [w321 w323 w330] -> w310
              tunnel: w316 -> [w319 w323 w330]
              tunnel: w314 -> [w320 w324 w328]
              tunnel: [w317 w325 w327] -> w313
              frame "Measuring", Default {
                # "If the system is logging, stop logging."
                n107 = call "Pause.vi"("error in (no error)"=w319, "State in"=w320) -> ("error out"=w321:errorcluster, "State out"=w318:T18)  [unwired: 8 in]
                n108 = Bundle By Name(cluster=w318, "State"=State_Enum."Paused") -> (w317:T18)
              }
              frame "Idle" {
                # "The system is already idle. Ignore the \"Stop\" message."
                n109 = Bundle By Name(cluster=w324, "State"=State_Enum."Paused") -> (w325:T18)
              }
              frame "Paused" {
                n110 = Bundle By Name(cluster=w328, "State"=State_Enum."Paused") -> (w327:T18)
              }
            }
            n111 = call-poly "Enqueue Message.vi"("error in (no error)"=w310, "Message Data"=w308, "Message"="Update", "Message Queue"=w311) -> ("error out"=w309:errorcluster)  [unwired: 6 in, 1 out]
          }
          frame "Update Settings" {
            # "New settings are available, update the current ones stored in the shift register with the settings sent as part of the message"
            n112 = Variant To Data(error in=w339, type=T9 {"GUID"="", "Drop Coords"={"Horizontal"=0, "Vertical"=0}, "Process Name"="", "Queue Name"="", "Settings"={"Cycle Period"=0.0, "Setpoint Entry"=0.0, "Output Device"=enum."Default", "Huber Ministat 230 Settings"={"VISA resource name"="", "Simulated?"=FALSE}, "Lauda Settings"={"VISA resource name"="", "Simulated?"=FALSE, "Pump Power"=2}, "Julabo FP-50 Settings"={"VISA resource name"="", "Simulated?"=FALSE, "Pump Power"=2}, "Internal Control?"=FALSE, "Huber Unistat 410 Settings"={"VISA resource name"="", "Simulated?"=FALSE}}, "Load Count"=0, "Power Level Changed"=FALSE} ("TCU Module Config Out"), Variant=w340) -> (data=w333:T9, error out=w335:errorcluster)
            n113 = Unbundle By Name(w333) -> ("Settings"=w331:T11, "Power Level Changed"=w332:bool)
            n114 = Bundle By Name(cluster=w337, "Configuration"=w331, "Power Level Changed"=w332) -> (w336:T18)
          }
          frame "Exit" {
            # "Release the Logging queue reference"
            # "Don't check the error out. The UI message queue may have already been released."
            # "Stop the VI"
            # "Exit - Send the Exit message to the UI Message Handler.  Call 'Flush Data to Log File.vi' so any pending data is not lost."
            n115 = Release Queue(queue=w345, error in (no error)=w348) -> (error out=w344:errorcluster)  [unwired: 1 in, 2 out]
            n116 = call-poly "Enqueue Message.vi"("Priority Message? (F)"=TRUE, "Message"="Exit", "Message Queue"=w349) -> ("error out"=w342:errorcluster)  [unwired: 7 in, 1 out]
            n117 = call <vilib>:"Clear Errors.vi"("error in (no error)"=w342) -> ()  [unwired: 5 in, 2 out]
            n118 = Merge Errors(w344) -> (w350:errorcluster)
          }
          frame "---Copy This Frame---" {
            # "Duplicate this frame when creating new messages.  Change this comment in the duplicated frame to describe this message."
            n119 = Merge Errors(w355) -> (w353:errorcluster)
          }
          frame "Initialize" {
            # "Reset First Iteration and Start Log"
            n120 = Merge Errors(w362) -> (w361:errorcluster)
            n121 = Bundle By Name(cluster=w359, "First Iteration"=TRUE, "Start Log"=FALSE) -> (w356:T18)
          }
          frame Default {
            # "'Default' case only runs if there is a message that isn't defined in any of the other cases.  Output a programming error."
            n122 = Concatenate Strings("The invalid message string " ("string"), w363, " was received in the TCU Module Engine." ("string")) -> (w365:string)
            n123 = Bundle By Name(cluster=errorcluster {"status"=TRUE, "code"=1, "source"=""} ("error constant"), "source"=w365) -> (w364:errorcluster)
          }
        }
        n124 = Unbundle By Name(w27) -> ("State"=w26:T8, "Configuration.Cycle Period"=w24:dbl)
        n125 = call "Error Handler.vi"("error in (no error)"=w33, "Message Queue"=w31) -> ("dup error in"=w32:errorcluster)  [unwired: 8 in, 1 out]
        n126 = case shown="\"Measuring\"" w26 {
          tunnel: [w41 1 1] -> w25
          tunnel: w24 -> [w41 _ _]
          frame "Measuring" {
          }
          frame "Idle" {
          }
          frame "Paused" {
          }
        }
        n127 = node-c288(w25) -> ()  [unwired: 1 in, 1 out]
      }
      n128 = node-c288(w11) -> ()  [unwired: 1 out]
    }
    frame Error {
    }
  }
  "error out" <- w3
